vi "Limelight Distance.vi"() -> (2 "x/y":dbl)   [LabVIEW 2019]
uses:
  <vilib>/Rock Robotics/Network Tables/NT Read Number.vi
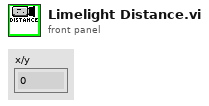
[diagram p1: front panel]
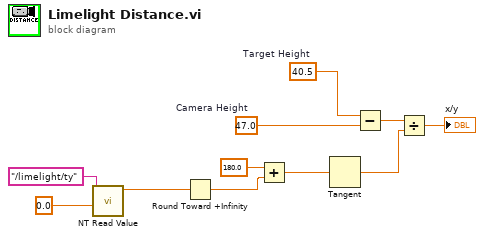
[diagram p0: block diagram]
diagram:
  w2 = 40.5  # Target Height
  w3 = 47.0  # Camera Height
  n1 = call-poly <vilib>:"NT Read Value.vi"("Default Value"=0.0, "Name"="/limelight/ty") -> ("Numeric"=w9:dbl)  [unwired: 8 in, 1 out]
  n2 = Round Toward +Infinity(x=w9) -> (ceil(x): smallest int >= x=w8:dbl)
  n3 = Add(x=180.0, y=w8) -> (x+y=w6:dbl)
  n4 = Tangent(1:w6) -> (0:w5:dbl)
  n5 = Subtract(x=w2, y=w3) -> (x-y=w4:dbl)
  n6 = Divide(x=w4, y=w5) -> (x/y=→"x/y":dbl)
